vi "making class not screw up.vi"() -> (0 "max jitter (uS)":dbl format="%.2f", 1 "mean time (uS)":dbl format="%.2f", 2 "standard deviation (uS)":dbl format="%.2f", 3 "execution histogram":T1(graph), 4 "Error":errorcluster, 5 "execution times (uS)":dbl[](graph))   [LabVIEW 2013]
uses:
  <vilib>/platform/TimedLoop/XDataNode/XDataNode.xnode
  <vilib>/Platform/TimedLoop/XDataNode/nitl_modes.ctl
  <vilib>/Platform/TimedLoop/XDataNode/XDNodeRunTimeDep.lvlib
  <vilib>/Platform/TimedLoop/XDataNode/wakeup.ctl
  <vilib>/Platform/TimedLoop/XDataNode/timing_clust.ctl
panel:
  out "act start":timestamp
  out "current time":timestamp
  out "start":timestamp
  out "actual":dbl format="%#_32f"
  out "desired":dbl format="%#_32f"
  out "diff":dbl format="%#_32f"
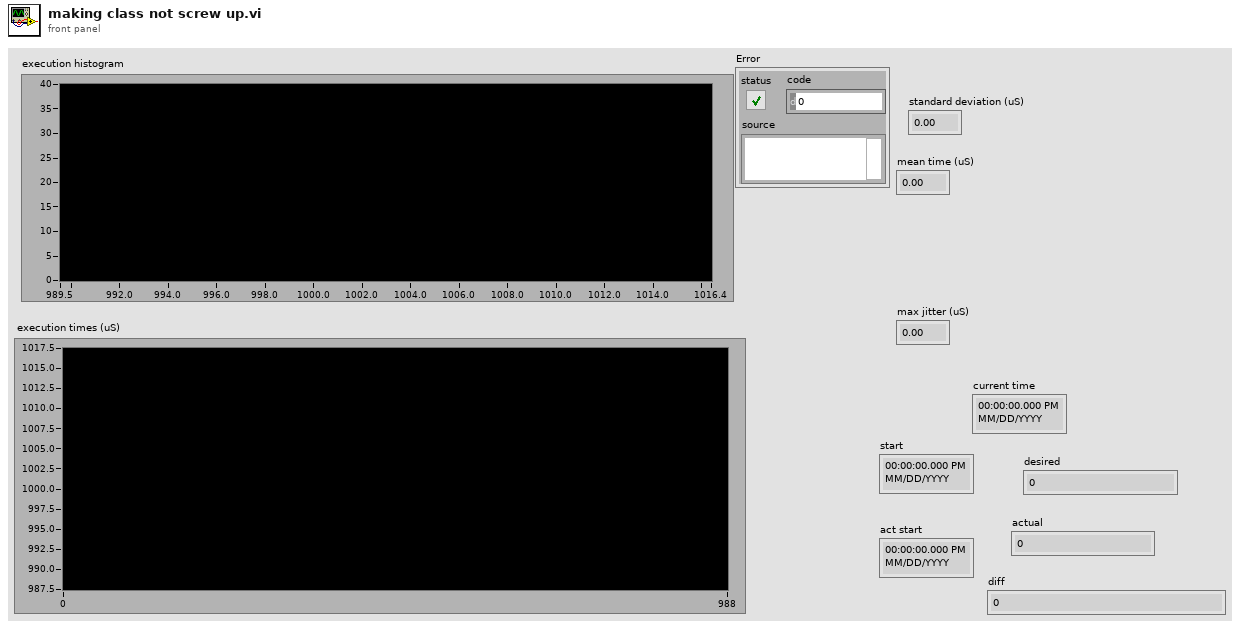
[diagram p1: front panel]
types:
  T1 = cluster{"X Values":dbl[], "Histogram: h(x)":i32[]}
  T2 = typedef "XDNodeRunTimeDep.lvlib/timing_clust.ctl" = cluster{"Expected End [f-1]":u64, "Actual End [f-1]":u64, "Finished Late? [f-1]":bool, "Expected End [i-1]":u64, "Actual End [i-1]":u64, "Finished Late? [i-1]":bool, "Expected Start [i]":u64, "Actual Start [i]":u64, "Expected Start [f]":u64, "Actual Start [f]":u64, "Source Name":string, "Structure Name":string, "Period":i64, "Deadline":i64, "Offset":i64, "Start":i64, "Priority":i32, "Timeout":i32, "Mode":T3, "Wakeup Reason":T4, "Error":errorcluster, "Source Type":string, "Secondary Source Type":string, "Global End Time":u64, "Global Start Time":u64, "Frame Duration":u64, "Iteration Duration":u64, "Assigned CPU":i32, "I/O Scan Engine Mode":u32}
  T3 = typedef "XDNodeRunTimeDep.lvlib/nitl_modes.ctl" = enum32{"No Change", "Process missed periods, maintain original phase", "Discard missed periods, maintain original phase", "Process missed periods, ignore original phase", "Discard missed periods, ignore original phase"}
  T4 = typedef "XDNodeRunTimeDep.lvlib/wakeup.ctl" = enum32{"Normal", "Aborted", "Asynchronous wakeup", "Timing source error", "Timed loop error", "Timeout"}
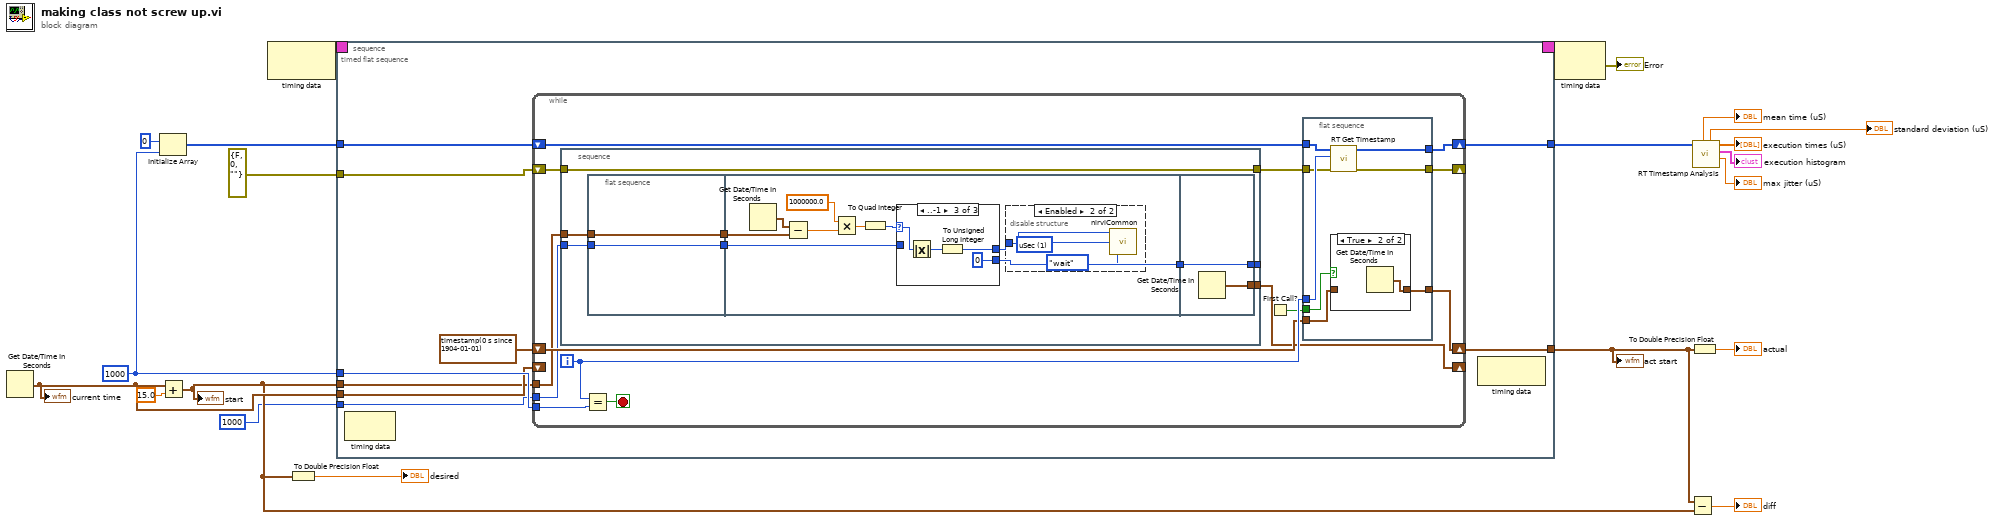
[diagram p0: block diagram]
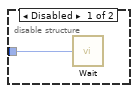
[diagram p2: hidden frame]
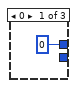
[diagram p3: hidden frame]
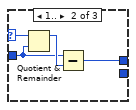
[diagram p4: hidden frame]
diagram:
  w19 = 1000 ("x")
  n1 = Get Date/Time In Seconds() -> (seconds since 1Jan1904=w4:timestamp)
  "current time" <- w4
  n2 = Initialize Array(u64 0, w19) -> (w20:u64[])
  n3 = Add(x=w4, y=15.0) -> (x+y=w3:timestamp)
  "start" <- w3
  n4 = node-c288() -> (w12:T2)  [unwired: 1 in]
  n5 = To Double Precision Float(number=w3) -> (double precision float=→"desired":dbl)
  n6 = timed-sequence {
    timing: w12 -> [_]
    timing-out: [_] -> w11
    tunnel: w19 -> [w29]
    tunnel: w20 -> [w28]
    tunnel: [w27] -> w18
    tunnel: errorcluster {"status"=FALSE, "code"=0, "source"=""} ("error out") -> [w26]
    tunnel: [w25] -> w6
    tunnel: w4 -> [w24]
    tunnel: w3 -> [w23]
    tunnel: u32 1000 ("dt") -> [w22]
    n7 = timed-flat-sequence {
      tunnel: w29 -> [w38]
      tunnel: w28 -> [w37]
      tunnel: [w36] -> w27
      tunnel: w26 -> [w35]
      tunnel: [w33] -> w25
      tunnel: w24 -> [w32]
      tunnel: w23 -> [w31]
      tunnel: w22 -> [w30]
      n8 = node-c288() -> ()  [unwired: 1 in, 1 out]
      n9 = while {
        tunnel: w38 -> [w52]
        shift-right: [w50] -> w36
        shift-left: w37 -> [w51]
        shift-right: [w46] -> _
        shift-left: w35 -> [w45]
        shift-right: [w43] -> w33
        shift-left: timestamp(0 s since 1904-01-01) ("seconds since 1Jan1904") -> [w42]
        shift-right: [w41] -> _
        shift-left: w32 -> [_]
        tunnel: w31 -> [w40]
        tunnel: w30 -> [w39]
        i -> [w48]
        stop <- w49 stop-if-true
        n10 = stacked-sequence {
          tunnel: [w58] -> w47
          tunnel: [w59] -> _
          tunnel: w45 -> [w58]
          tunnel: [w57] -> w41
          tunnel: w40 -> [w56]
          tunnel: w39 -> [w55]
          frame #0 {
            n11 = flat-sequence {
              tunnel: w56 -> [w61]
              tunnel: w55 -> [w62]
              tunnel: [w62] -> w54
              tunnel: [w61] -> w53
              tunnel: [w65] -> w60
              tunnel: w54 -> [w66]
              tunnel: w53 -> [w64]
              tunnel: [w86] -> w59
              tunnel: w60 -> [w86]
              tunnel: [w85] -> w57
              frame #0 {
              }
              frame #1 {
                n12 = Get Date/Time In Seconds() -> (seconds since 1Jan1904=w71:timestamp)
                n13 = Subtract(x=w71, y=w64) -> (x-y=w70:dbl)
                n14 = Multiply(x=1000000.0, y=w70) -> (x*y=w68:dbl)
                n15 = To Quad Integer(1:w68) -> (0:w67:i64)
                n16 = case shown="..-1" w67 {
                  selector: w67 -> [_ w80 w84]
                  tunnel: w66 -> [_ w78 _]
                  tunnel: [u32 0 w77 w81] -> w63
                  tunnel: [_ _ u32 0] -> w65
                  frame 0 {
                  }
                  frame 1.. {
                    n17 = Quotient & Remainder(x=w80, y=w78) -> (x-y*floor(x/y)=w79:i64)  [unwired: 1 out]
                    n18 = Subtract(x=w78, y=w79) -> (x-y=w77:u32)
                  }
                  frame ..-1 {
                    n19 = Absolute Value(x=w84) -> (abs(x)=w83:i64)
                    n20 = To Unsigned Long Integer(number=w83) -> (unsigned 32bit integer=w81:u32)
                  }
                }
                n21 = disable-structure shown="Enabled" {
                  disable-tunnel: w63 -> [w72 w73]
                  frame Disabled {
                    n22 = call "Wait"("Count(uSec)"=w72) -> ()  [unwired: 1 out]
                  }
                  frame Enabled {
                    w74 = u16 1 items=["Ticks", "uSec", "mSec"] ("Counter Units")
                    n23 = call <vilib>:"nirviCommon.vi"("Action"=enum16{"wait", "wait multiple", "tick count"}."wait", "Counter Units"=w74, "Count(uSec)"=w73) -> ()  [unwired: 1 out]
                  }
                }
              }
              frame #2 {
                n24 = Get Date/Time In Seconds() -> (seconds since 1Jan1904=w85:timestamp)
              }
            }
          }
        }
        n25 = Equal?(x=w48, y=w52) -> (x = y?=w49:bool)
        n26 = First Call?() -> (First Call?: T/F=w44:bool)
        n27 = flat-sequence {
          tunnel: w51 -> [w94]
          tunnel: [w93] -> w50
          tunnel: w48 -> [w92]
          tunnel: w47 -> [w91]
          tunnel: [w90] -> w46
          tunnel: w44 -> [w89]
          tunnel: [w88] -> w43
          tunnel: w42 -> [w87]
          frame #0 {
            n28 = call <vilib>:"RT Get Timestamp.vi"("error in (no error)"=w91, "iteration"=w92, "timestamp array in"=w94) -> ("error out"=w90:errorcluster, "timestamp array out"=w93:u64[])  [unwired: 7 in]
            n29 = case shown="True" w89 {
              tunnel: [w95 w96] -> w88
              tunnel: w87 -> [w95 _]
              frame False {
              }
              frame True {
                n30 = Get Date/Time In Seconds() -> (seconds since 1Jan1904=w96:timestamp)
              }
            }
          }
        }
      }
      n31 = node-c288() -> ()  [unwired: 1 in, 1 out]
    }
  }
  "act start" <- w6
  n32 = node-c288(w11) -> (→"Error":errorcluster)
  n33 = Subtract(x=w6, y=w3) -> (x-y=→"diff":dbl)
  n34 = To Double Precision Float(number=w6) -> (double precision float=→"actual":dbl)
  n35 = call <vilib>:"RT Timestamp Analysis.vi"("timestamp array"=w18) -> ("max jitter (uS)"=→"max jitter (uS)":dbl, "execution histogram"=→"execution histogram":T1, "execution times (uS)"=→"execution times (uS)":dbl[], "standard deviation (uS)"=→"standard deviation (uS)":dbl, "mean time (uS)"=→"mean time (uS)":dbl)  [unwired: 5 in, 1 out]
